vi "HW Init Outcome.vi"(8 "error in (no error)":errorcluster, 10 "Outcome":T2) -> (0 "error out":errorcluster)   [LabVIEW 2018, in "HW Interaction.lvlib"]
doc: "Broadcasts the outcome of the HW Init sequence.\n_____\nCreated using Delacor QMH Event Scripter 4.2.1.88."
uses:
  HW Interaction.lvlib
  Public API/Typedefs/CTL_Sensor_board_type_(size).ctl
  HW Init Outcome Argument--cluster.ctl
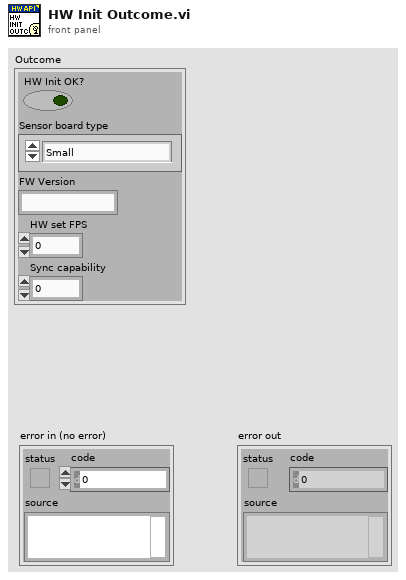
[diagram p1: front panel]
types:
  T1 = typedef "HW Interaction.lvlib/CTL_Sensor_board_type_(size).ctl" = enum16{"Small", "Large"}
  T2 = cluster{"HW Init OK?":bool, "Sensor board type":T1, "FW Version":string, "HW set FPS":dbl, "Sync capability":u8}
  T3 = typedef "HW Interaction.lvlib/HW Init Outcome Argument--cluster.ctl" = cluster{"Outcome":cluster{"HW Init OK?":bool, "Sensor board type":T1, "FW Version":string, "HW set FPS":dbl, "Sync capability":u8}}
  T4 = typedef "HW Interaction.lvlib/Broadcast Events--cluster.ctl" = cluster{"Module Did Init":refnum<user-event>, "Status Updated":refnum<user-event>, "Error Reported":refnum<user-event>, "Module Did Stop":refnum<user-event>, "Update Module Execution Status":refnum<user-event>, "HW Init Outcome":refnum<user-event>}
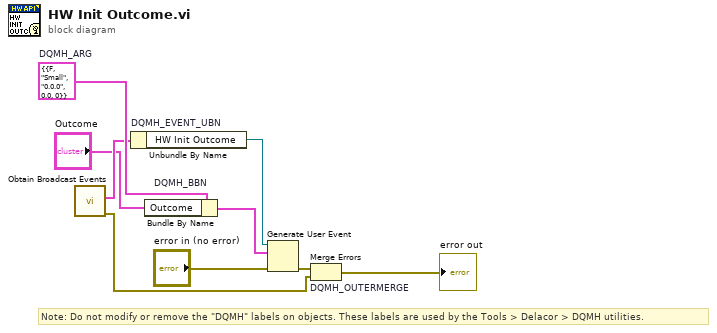
[diagram p0: block diagram]
diagram:
  w4 = T3 {"Outcome"={"HW Init OK?"=FALSE, "Sensor board type"=enum."Small", "FW Version"="0.0.0", "HW set FPS"=0.0, "Sync capability"=0}}  # DQMH_ARG
  # "Note: Do not modify or remove the \"DQMH\" labels on objects. These labels are used by the Tools > Delacor > DQMH utilities."
  n1 = call "Obtain Broadcast Events.vi"() -> ("error out"=w3:errorcluster, "HW Interaction Broadcast Events"=w2:T4)  [unwired: 10 in]
  n2 = Unbundle By Name "DQMH_EVENT_UBN"(w2) -> ("HW Init Outcome"=w6:refnum<user-event>)
  n3 = Bundle By Name "DQMH_BBN"(cluster=w4, "Outcome"="Outcome") -> (w7:T3)
  n4 = Generate User Event(user event=w6, event data cluster=w7, error in="error in (no error)") -> (error out=w5:errorcluster)  [unwired: 1 in, 1 out]
  n5 = Merge Errors "DQMH_OUTERMERGE"(w5, w3) -> (→"error out":errorcluster)
